vi "Initialise cRIO.vi"(7 "error in":errorcluster) -> (13 "Shutdown Notifier":refnum<notifier>, 15 "Emergency Turn Off Notifier":refnum<notifier>, 19 "Update Motors Notifier":refnum<notifier>, 20 "Log File Cluster":T1, 21 "CANOpen Session":refnum<k20>, 22 "CAN Session":T3, 26 "Error Queue":refnum<queue>, 27 "error out":errorcluster)   [LabVIEW 2016]
uses:
  Program Files (x86)/National Instruments/LabVIEW 2016/examples/robotics/EPOS2 CANOpen Driver/Low Level VIs/Typedefs/CAN Refnum.ctl
  Program Files (x86)/National Instruments/LabVIEW 2016/examples/robotics/EPOS2 CANOpen Driver/Low Level VIs/Typedefs/CAN Session Pointer.ctl
  Program Files (x86)/National Instruments/LabVIEW 2016/examples/robotics/EPOS2 CANOpen Driver/Low Level VIs/Typedefs/CAN Communication References.ctl
  Program Files (x86)/National Instruments/LabVIEW 2016/examples/robotics/EPOS2 CANOpen Driver/Low Level VIs/Typedefs/kill process notifier array.ctl
  Program Files (x86)/National Instruments/LabVIEW 2016/examples/robotics/EPOS2 CANOpen Driver/Low Level VIs/Typedefs/Write Queue.ctl
  Program Files (x86)/National Instruments/LabVIEW 2016/examples/robotics/EPOS2 CANOpen Driver/Low Level VIs/Typedefs/FPGA CAN Frame Cluster.ctl
  Tests/Log File Cluster.ctl
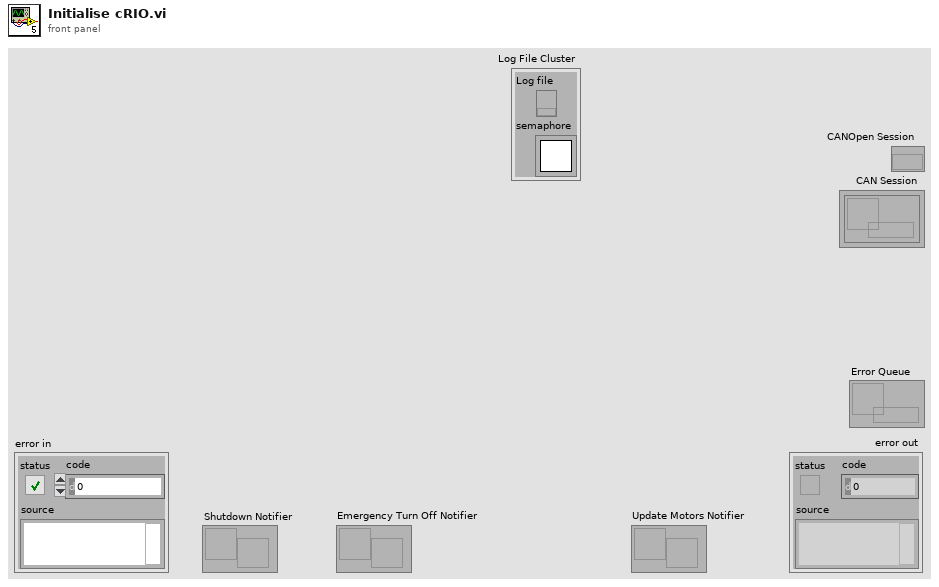
[diagram p1: front panel]
types:
  T1 = typedef "Log File Cluster.ctl" = cluster{"Log file":refnum<k34>, "semaphore":T2}
  T2 = typedef "Semaphore RefNum" = refnum<k1>
  T3 = typedef "CAN Refnum.ctl" = refnum<k1>
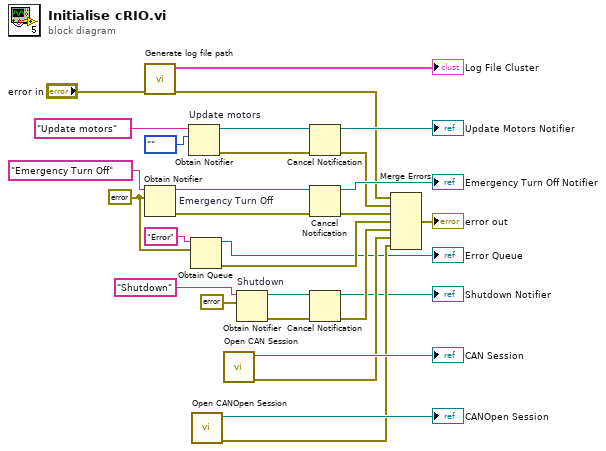
[diagram p0: block diagram]
diagram:
  w4 = errorcluster {"status"=FALSE, "code"=0, "source"=""} ("error constant")
  n1 = call "Generate log file path.vi"("error in"="error in") -> ("error out"=w19:errorcluster, "Log File Cluster"=→"Log File Cluster":T1)  [unwired: 9 in]
  n2 = Obtain Notifier "Emergency Turn Off"(name (unnamed)="Emergency Turn Off", notification data type=w4) -> (notifier out=w28:refnum<notifier>, error out=w26:errorcluster)  [unwired: 2 in, 1 out]
  n3 = Obtain Notifier "Update motors"(name (unnamed)="Update motors", notification data type=enum16{""}."") -> (notifier out=w24:refnum<notifier>, error out=w25:errorcluster)  [unwired: 2 in, 1 out]
  n4 = Obtain Queue(name (unnamed)="Error", element data type=w4) -> (queue out=→"Error Queue":refnum<queue>, error out=w3:errorcluster)  [unwired: 3 in, 1 out]
  n5 = call "Open CANOpen Session.vi"() -> ("error out"=w15:errorcluster, "interface object out"=→"CANOpen Session":refnum<k20>)  [unwired: 10 in]
  n6 = call "Open CAN Session.vi"() -> ("error out"=w16:errorcluster, "CAN Session"=→"CAN Session":T3)  [unwired: 10 in]
  n7 = Obtain Notifier "Shutdown"(name (unnamed)="Shutdown", notification data type=errorcluster {"status"=FALSE, "code"=0, "source"=""} ("error constant")) -> (notifier out=w8:refnum<notifier>, error out=w13:errorcluster)  [unwired: 2 in, 1 out]
  n8 = Cancel Notification(0:w24, 3:w25) -> (8:→"Update Motors Notifier":refnum<notifier>, 11:w18:errorcluster)  [unwired: 1 out]
  n9 = Cancel Notification(0:w28, 3:w26) -> (8:→"Emergency Turn Off Notifier":refnum<notifier>, 11:w17:errorcluster)  [unwired: 1 out]
  n10 = Cancel Notification(0:w8, 3:w13) -> (8:→"Shutdown Notifier":refnum<notifier>, 11:w7:errorcluster)  [unwired: 1 out]
  n11 = Merge Errors(w19, w18, w17, w3, w7, w16, w15) -> (→"error out":errorcluster)
